vi "template_Job (JKI-SM).vi"() -> ()   [LabVIEW 2013]
doc: "Job template based on the popular JKI State Machine."
uses:
  <vilib>/LabVIEW Open Source Project/Cron Scheduler/Job/Job.lvclass
  <vilib>/LabVIEW Open Source Project/Cron Scheduler/Job/Job.lvclass/Job.ctl
  <vilib>/LabVIEW Open Source Project/Cron Scheduler/Job/Read Abort Notifier.vi
panel:
  out "Job out":refnum<class "Job.lvclass">
  out "error out":errorcluster
  in  "Job":refnum<class "Job.lvclass">
  out "stdout":string
  in  "stdin":string
  # "Macro: Initialize\nList the tasks to be execute for this job\n\nThere are two ways to terminate the job: \n1- Call the \"Macro: Exit\" state at the end of your task execution.\n2- Comment out the \"Macro: Exit\" state in \"Macro: Initialize\" case and monitor a Job completion condition instead. Use the \"Action: Check Job Complete\" state to instruct the job to terminate.\n\nAction: Read Standard Input\nUse this case to read the stdin terminal and initialize your job.\n\nAction: Write Standard Output\nMake sure to write your return value to the stdout terminal before exiting this VI."
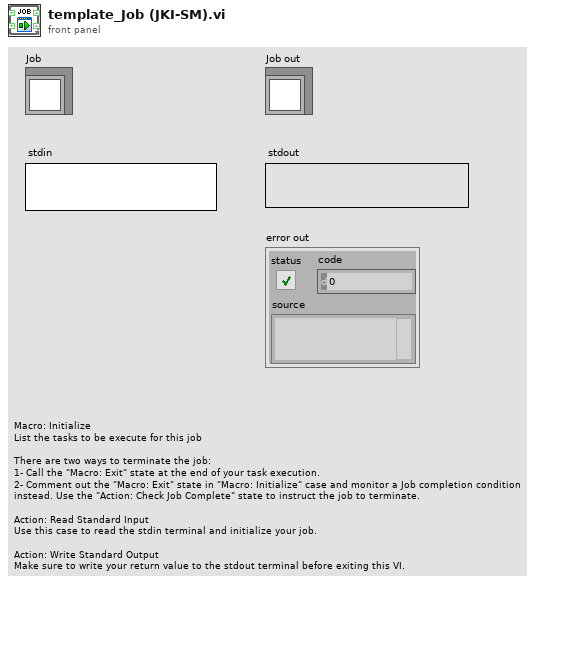
[diagram p1: front panel]
types:
  T1 = enum32{"Invalid", "Standard", "Closed", "Hidden", "Minimized", "Maximized"}
  T2 = enum32{"invalid app kind", "Development System", "Run Time System", "Student Edition", "Embedded LabVIEW", "Evaluation", "Custom"}
  T3 = cluster{"Core":cluster{"Current VI Reference":refnum<vi>, "Close Panel on Exit?":bool}, "Job":refnum<class "Job.lvclass">, "stdin":string, "stdout":string, "stderror":errorcluster, "start time":timestamp}
  T4 = cluster{"Current VI Reference":refnum<vi>, "Close Panel on Exit?":bool}
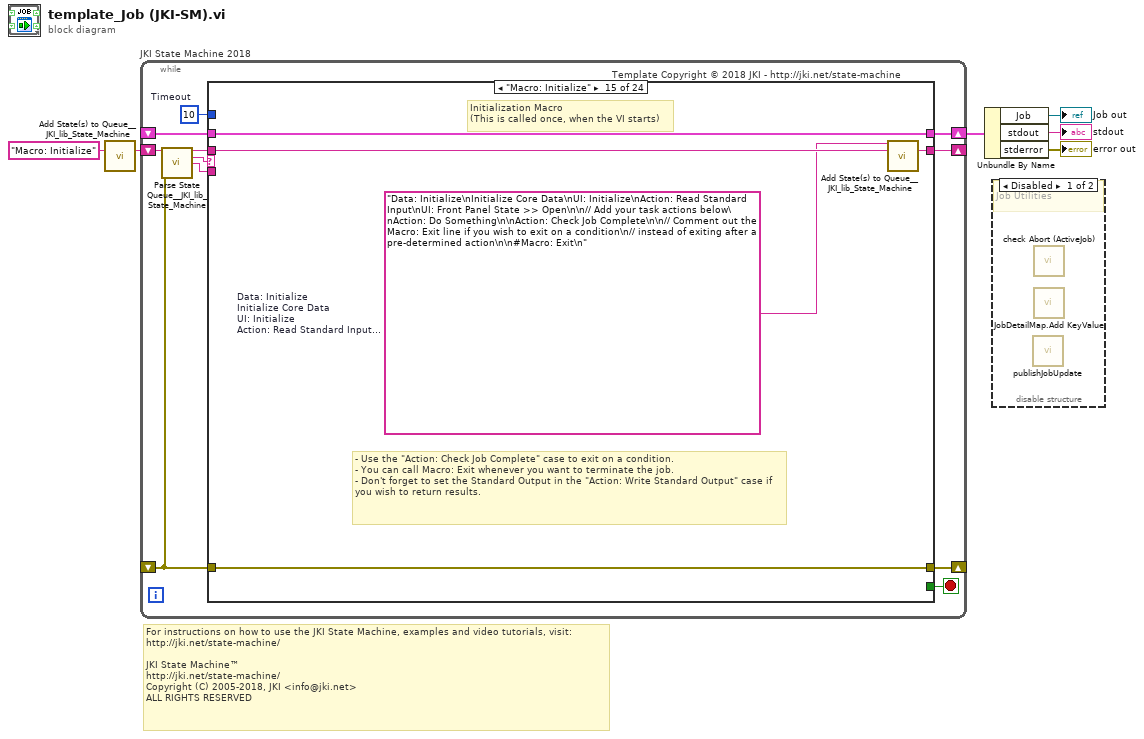
[diagram p0: block diagram]
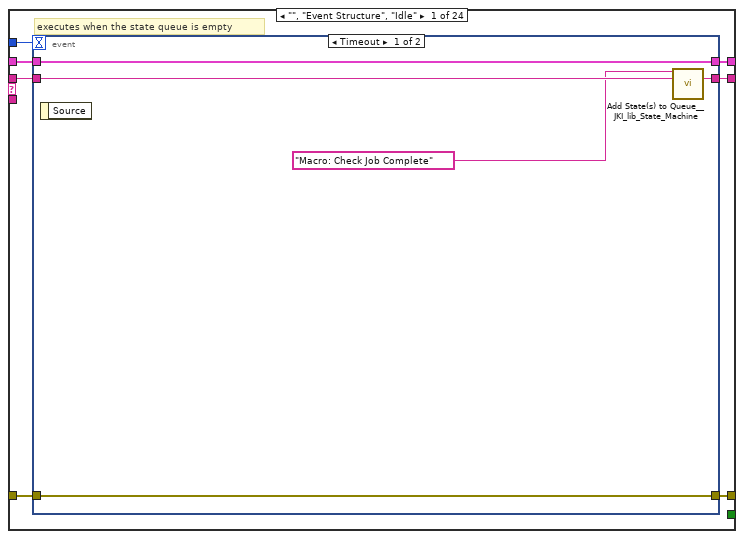
[diagram p3: hidden frame]
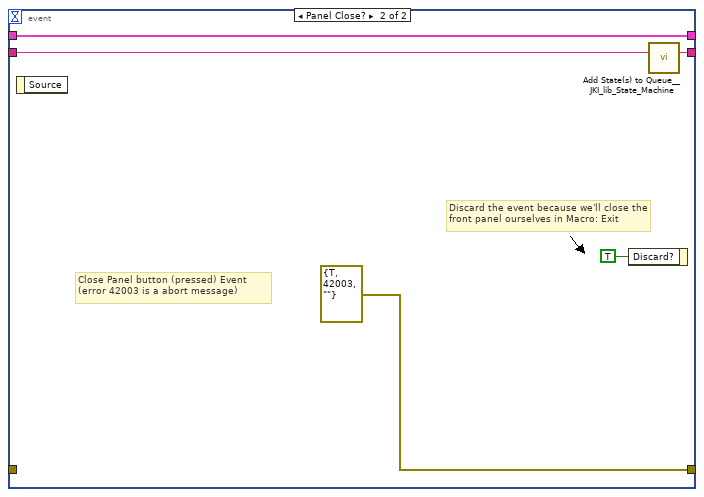
[diagram p4: hidden frame]
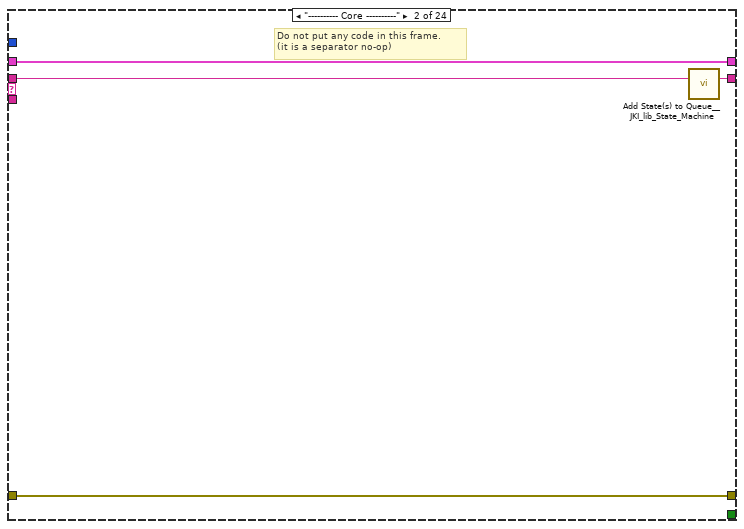
[diagram p5: hidden frame]
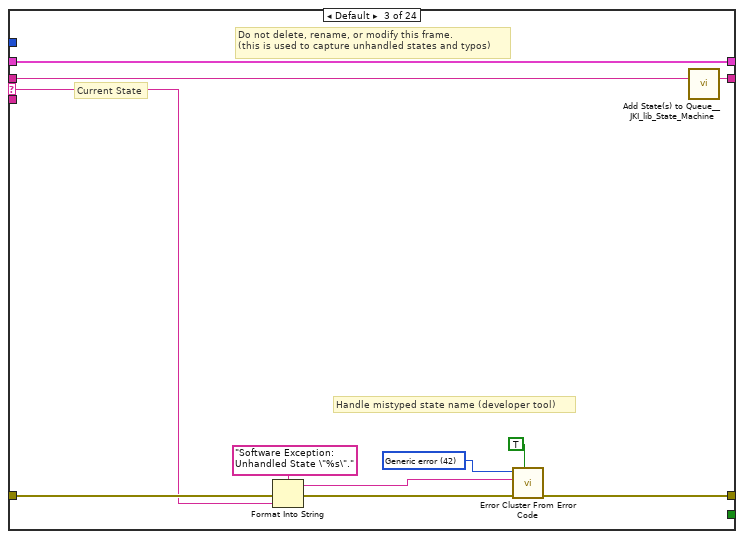
[diagram p6: hidden frame]
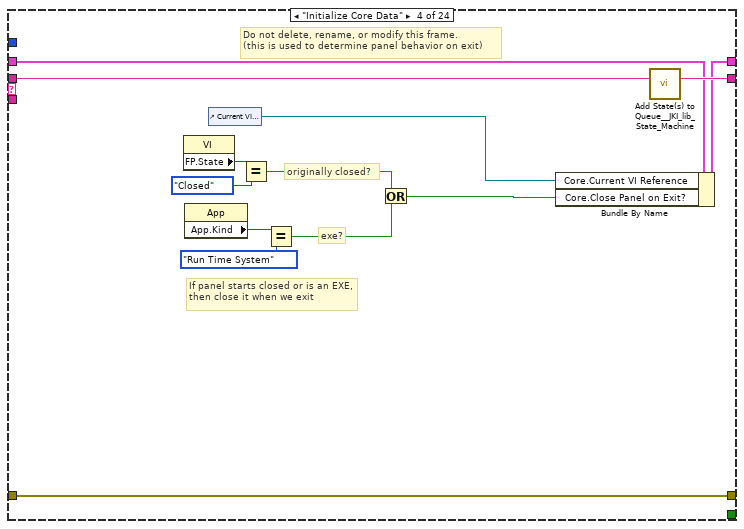
[diagram p7: hidden frame]
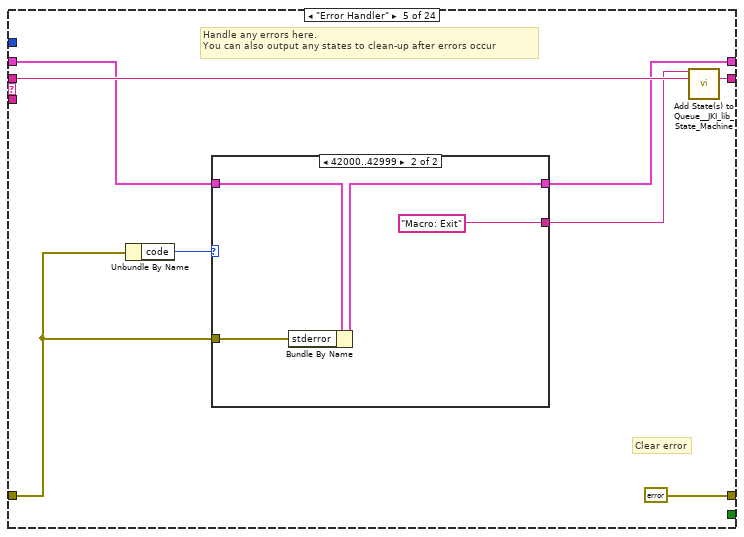
[diagram p8: hidden frame]
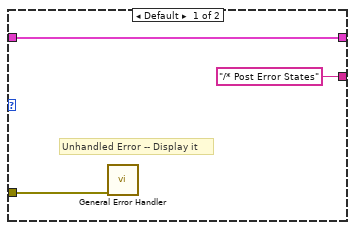
[diagram p9: hidden frame]
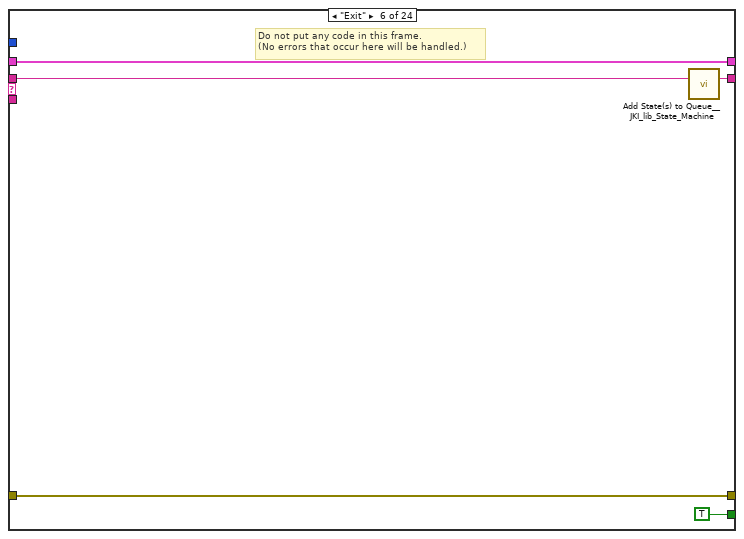
[diagram p10: hidden frame]
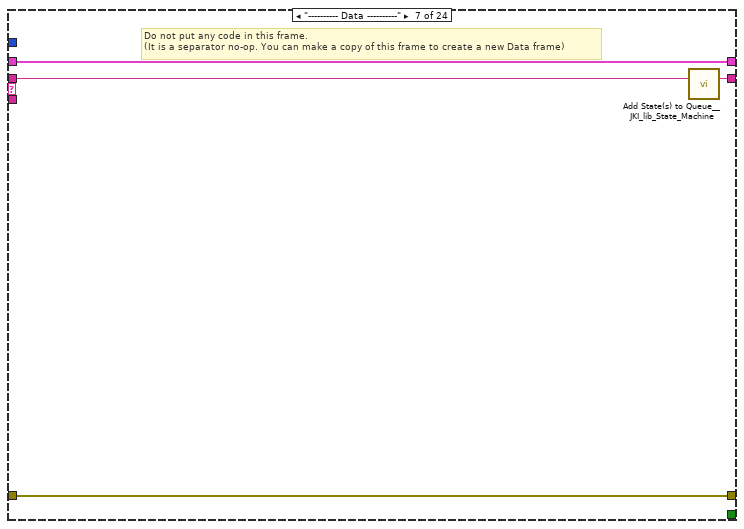
[diagram p11: hidden frame]
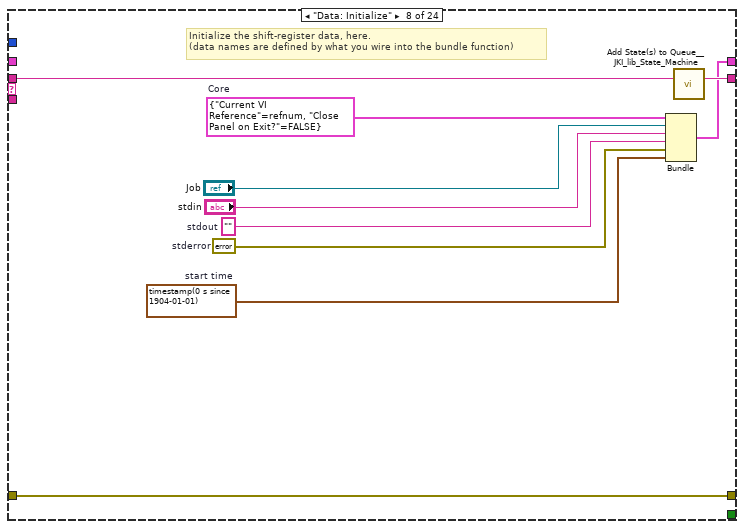
[diagram p12: hidden frame]
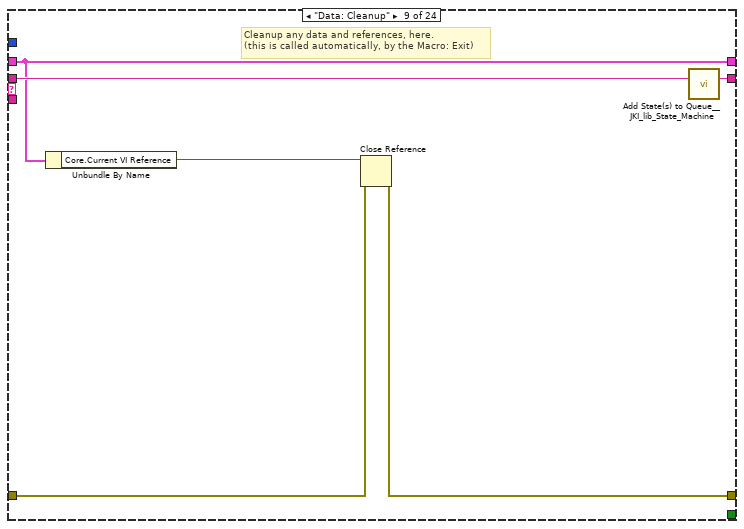
[diagram p13: hidden frame]
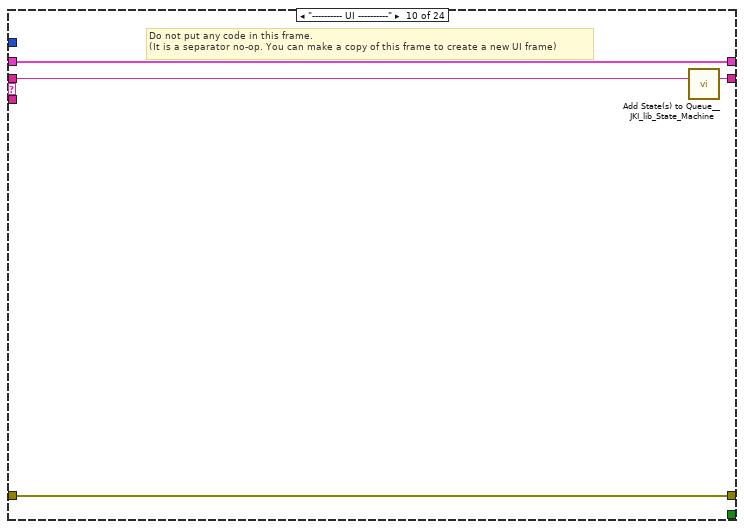
[diagram p14: hidden frame]
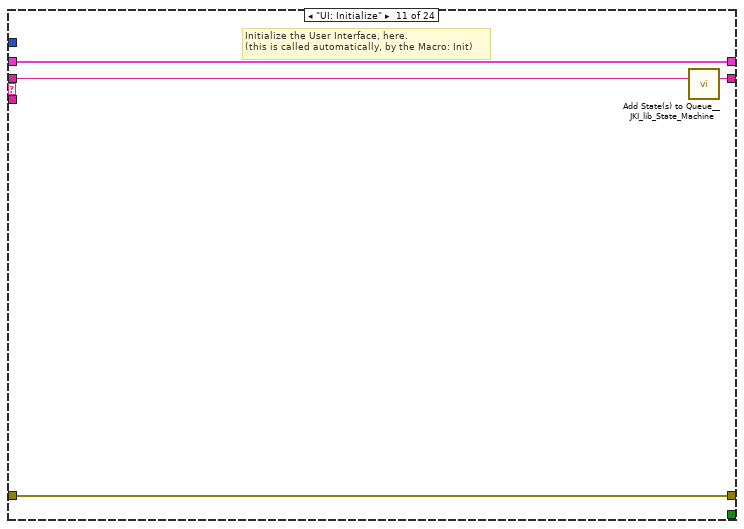
[diagram p15: hidden frame]
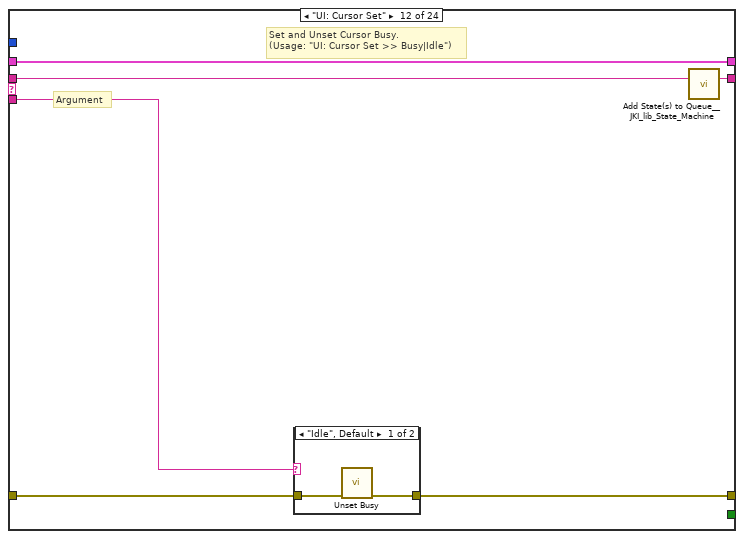
[diagram p16: hidden frame]
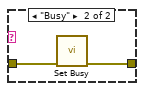
[diagram p17: hidden frame]
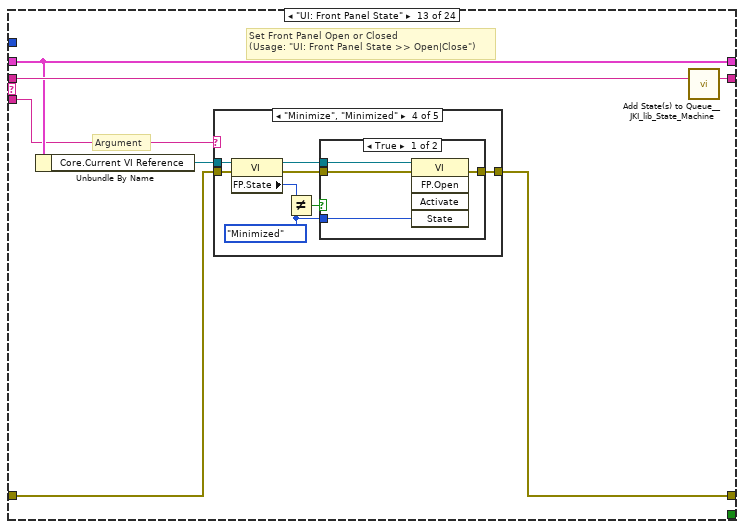
[diagram p18: hidden frame]
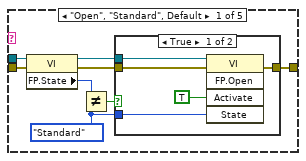
[diagram p19: hidden frame]
diagram:
  # "For instructions on how to use the JKI State Machine, examples and video tutorials, visit:\nhttp://jki.net/state-machine/\n\nJKI State Machine™\nhttp://jki.net/state-machine/\nCopyright (C) 2005-2018, JKI <info@jki.net>\nALL RIGHTS RESERVED"
  n1 = call <vilib>:"Add State(s) to Queue__JKI_lib_State_Machine.vi"("State(s) in (\"\")"="Macro: Initialize") -> ("States Out"=w6:string)  [unwired: 14 in]
  n2 = while "JKI State Machine 2018" {
    shift-right: [w10] -> w4
    shift-left: _ -> [w9]
    shift-right: [w13] -> _
    shift-left: _ -> [w7]
    shift-right: [w12] -> _
    shift-left: w6 -> [w14]
    stop <- w11 stop-if-true
    w8 = 10  # Timeout
    # "Template Copyright © 2018 JKI - http://jki.net/state-machine"
    n3 = call <vilib>:"Parse State Queue__JKI_lib_State_Machine.vi"("State Queue"=w14, "Error In (no error)"=w7) -> ("Remaining States"=w16:string, "Current State"=w17:string, "Arguments"=w15:string)  [unwired: 11 in]
    n4 = case shown="\"Macro: Initialize\"" w17 {
      selector: w17 -> [_ _ w39 _ _ _ _ _ _ _ _ _ _ _ _ _ _ _ w230 _ _ _ _ _]
      tunnel: w16 -> [w24 w38 w43 w62 w70 w82 w86 w96 w102 w106 w110 w116 w127 w196 w201 w206 w217 w223 w236 w251 w261 w271 w277 w288]
      tunnel: w15 -> [_ _ _ _ _ _ _ _ _ _ _ w111 w121 _ _ _ _ _ _ _ _ _ _ _]
      tunnel: w9 -> [w22 w35 w41 w55 w65 w80 w83 _ w97 w103 w108 w114 w123 w193 w198 w203 w214 w220 w234 w243 w259 w269 w273 w280]
      tunnel: [w21 w36 w45 w59 errorcluster {"status"=FALSE, "code"=0, "source"=""} ("error out") w79 w84 w93 w98 w104 w107 w112 w124 w194 w199 w204 w215 w221 w225 w249 w255 w263 w275 w286] -> w13
      tunnel: w7 -> [w20 w36 w44 w59 w66 w79 w84 w93 w99 w104 w107 w113 w125 w194 w199 w204 w215 w221 w231 w249 w252 w264 w275 w286]
      tunnel: [w23 w37 w42 w61 w69 w81 w85 w95 w101 w105 w109 w115 w126 w195 w200 w205 w216 w222 w235 w250 w260 w270 w276 w287] -> w12
      tunnel: [_ _ _ _ _ TRUE _ _ _ _ _ _ _ _ _ _ _ _ _ _ _ _ _ _] -> w11
      tunnel: [w19 w35 w41 w60 w64 w80 w83 w94 w97 w103 w108 w114 w123 w193 w198 w203 w214 w219 w233 w248 w258 w268 w272 w285] -> w10
      tunnel: w8 -> [w18 _ _ _ _ _ _ _ _ _ _ _ _ _ _ _ _ _ _ _ _ _ _ _]
      frame "", "Event Structure", "Idle" {
        # "executes when the state queue is empty"
        n5 = event shown="[0] Timeout" {
          selector: _ -> [_ _]
          dyn-events: _ -> [_ _]
          timeout: w18 -> [_ _]
          tunnel: w24 -> [w29 w34]
          tunnel: [w28 w33] -> w23
          tunnel: w22 -> [w26 w32]
          tunnel: [w27 errorcluster {"status"=TRUE, "code"=42003, "source"=""} ("error constant")] -> w21
          tunnel: w20 -> [w27 _]
          tunnel: [w26 w32] -> w19
          event Timeout {
            n6 = event-data() -> ()  [unwired: 1 in, 1 out]
            n7 = call <vilib>:"Add State(s) to Queue__JKI_lib_State_Machine.vi"("State(s) in Front (\"\")"="Macro: Check Job Complete", "State(s) in (\"\")"=w29) -> ("States Out"=w28:string)  [unwired: 13 in]
          }
          event Panel Close? {
            # "Discard the event because we'll close the front panel ourselves in Macro: Exit"
            # "Close Panel button (pressed) Event\n(error 42003 is a abort message)"
            n8 = event-data() -> ()  [unwired: 1 in, 1 out]
            n9 = event-data("Discard?"=TRUE) -> ()  [unwired: 1 in, 1 out]
            n10 = call <vilib>:"Add State(s) to Queue__JKI_lib_State_Machine.vi"("State(s) in (\"\")"=w34) -> ("States Out"=w33:string)  [unwired: 14 in]
          }
        }
      }
      frame "---------- Core ----------" {
        # "Do not put any code in this frame.\n(it is a separator no-op)"
        n11 = call <vilib>:"Add State(s) to Queue__JKI_lib_State_Machine.vi"("State(s) in (\"\")"=w38) -> ("States Out"=w37:string)  [unwired: 14 in]
      }
      frame Default {
        w48 = 42 items=["No error", "Argument error", "Memory is full", "Out of zone", "End of file", "File already open", "Generic file I/O error", "File not found", "File permission error", "Disk is full", "Duplicate path", "Too many files open", "System feature not enabled", "Resource file not found", "Cannot add resource", "Resource not found", "Image not found", "Image memory error", "Pen does not exist", "Config type invalid", "Config token not found", "Config parse error", "Config memory error", "Bad external code format", "Bad external code offset", "External code not present", "Null window", "Destroy window error", "Null menu", "Print aborted", "Bad print record", "Print driver error", "Windows error during printing", "Memory error during printing", "Print dialog error", "Generic print error", "Invalid device refnum", "Device not found", "Device parameter error", "Device unit error", "Cannot open device", "Device call aborted", "Generic error", "Cancelled by user", "Object ID too low", "Object ID too high", "Object not in heap", "Unknown heap", "Unknown object (invalid DefProc)", "Unknown object (DefProc not in table)", "Message out of range", "Invalid (null) method", "Unknown message", "Manager call not supported", "Bad address", "Network operation in progress", "Network operation timed out", "Connection is busy", "Network attribute not supported", "Network error", "Address in use", "System out of memory", "Connection aborted", "Connection refused", "Not connected", "Already connected", "Connection closed", "Initialization error (interapplication manager)", "Bad occurrence", "Wait on unbound occurrence handler", "Occurrence queue overflow", "Datalog type conflict", "Unused", "Unrecognized type (interapplication manager)", "Memory corrupt", "Failed to make temporary DLL", "Old CIN version", "Drag socket not found", "Failed to load drop-object", "Failed to register OLE object", "Failed to release OLE object", "Format specifier type mismatch", "Unknown format specifier", "Too few format specifiers", "Too many format specifiers", "Scan failed", "Newer CIN version", "Error converting to variant", "Runtime menu error", "Password tampered", "Variant attribute not found", "Incompatible variant data type", "Event data is not available", "Event Store is not present", "Occurrence is not found", "Event Queue is not created", "Event info is not available", "Refnum passed is NULL", "Error retrieving Class GUID", "Error retrieving CoClass GUID", "Error retrieving TypeLib GUID.", "Bad built application magic bytes.", "Specific driver is different from the specific driver associated with the Logical Name.", "There is no session opened to the class driver.", "Max Error", "MAX - Error with config objects", "MAX - Error loading configuration", "MAX - Group not supported"]
        # "Current State"
        # "Do not delete, rename, or modify this frame.\n(this is used to capture unhandled states and typos)"
        # "Handle mistyped state name (developer tool)"
        n12 = Format Into String(format string="Software Exception: Unhandled State \"%s\"." ("message"), error in=w44, w39) -> (resulting string=w47:string, error out=w46:errorcluster)  [unwired: 1 in]
        n13 = call <vilib>:"Error Cluster From Error Code.vi"("show call chain? (False)"=TRUE, "error in (no error)"=w46, "error message (\"\")"=w47, "error code (0)"=w48) -> ("error out"=w45:errorcluster)  [unwired: 5 in]
        n14 = call <vilib>:"Add State(s) to Queue__JKI_lib_State_Machine.vi"("State(s) in (\"\")"=w43) -> ("States Out"=w42:string)  [unwired: 14 in]
      }
      frame "Initialize Core Data" {
        # "Do not delete, rename, or modify this frame.\n(this is used to determine panel behavior on exit)"
        # "originally closed?"
        # "exe?"
        # "If panel starts closed or is an EXE, then close it when we exit"
        n15 = property class="VI"() -> ("FP.State"=w52:T1)  [unwired: 2 in, 2 out]
        n16 = property class="App"() -> ("App.Kind"=w58:T2)  [unwired: 2 in, 2 out]
        n17 = control-ref of="Current VI Reference"() -> (w53:refnum<vi>)
        n18 = Equal?(x=w52, y=T1."Closed" ("Front Panel Window:State")) -> (x = y?=w50:bool)
        n19 = Equal?(x=w58, y=T2."Run Time System" ("Application:Kind")) -> (x = y?=w56:bool)
        n20 = Or(x=w50, y=w56) -> (x .or. y?=w54:bool)
        n21 = Bundle By Name(cluster=w55, "Core.Current VI Reference"=w53, "Core.Close Panel on Exit?"=w54) -> (w60:T3)
        n22 = call <vilib>:"Add State(s) to Queue__JKI_lib_State_Machine.vi"("State(s) in (\"\")"=w62) -> ("States Out"=w61:string)  [unwired: 14 in]
      }
      frame "Error Handler" {
        # "Handle any errors here.\nYou can also output any states to clean-up after errors occur"
        # "Clear error"
        n23 = Unbundle By Name(w66) -> ("code"=w67:i32)
        n24 = case shown="42000..42999" w67 {
          tunnel: w66 -> [w73 w76]
          tunnel: w65 -> [w72 w77]
          tunnel: [w72 w75] -> w64
          tunnel: ["/* Post Error States" "Macro: Exit"] -> w63
          frame Default {
            # "Unhandled Error -- Display it"
            n25 = call <vilib>:"General Error Handler.vi"("error in (no error)"=w73) -> ()  [unwired: 10 in, 5 out]
          }
          frame 42000..42999 {
            n26 = Bundle By Name(cluster=w77, "stderror"=w76) -> (w75:T3)
          }
        }
        n27 = call <vilib>:"Add State(s) to Queue__JKI_lib_State_Machine.vi"("State(s) in Front (\"\")"=w63, "State(s) in (\"\")"=w70) -> ("States Out"=w69:string)  [unwired: 13 in]
      }
      frame "Exit" {
        # "Do not put any code in this frame.\n(No errors that occur here will be handled.)"
        n28 = call <vilib>:"Add State(s) to Queue__JKI_lib_State_Machine.vi"("State(s) in (\"\")"=w82) -> ("States Out"=w81:string)  [unwired: 14 in]
      }
      frame "---------- Data ----------" {
        # "Do not put any code in this frame.\n(It is a separator no-op. You can make a copy of this frame to create a new Data frame)"
        n29 = call <vilib>:"Add State(s) to Queue__JKI_lib_State_Machine.vi"("State(s) in (\"\")"=w86) -> ("States Out"=w85:string)  [unwired: 14 in]
      }
      frame "Data: Initialize" {
        w87 = timestamp(0 s since 1904-01-01)  # start time
        w88 = errorcluster {"status"=FALSE, "code"=0, "source"=""}  # stderror
        w89 = ""  # stdout
        w92 = T4 {"Current VI Reference"=refnum, "Close Panel on Exit?"=FALSE}  # Core
        # "Initialize the shift-register data, here.\n(data names are defined by what you wire into the bundle function)"
        n30 = Bundle("Core"=w92, "Job"="Job", "stdin"="stdin", "stdout"=w89, "stderror"=w88, "start time"=w87) -> (w94:T3)  [unwired: 1 in]
        n31 = call <vilib>:"Add State(s) to Queue__JKI_lib_State_Machine.vi"("State(s) in (\"\")"=w96) -> ("States Out"=w95:string)  [unwired: 14 in]
      }
      frame "Data: Cleanup" {
        # "Cleanup any data and references, here.\n(this is called automatically, by the Macro: Exit)"
        n32 = Unbundle By Name(w97) -> ("Core.Current VI Reference"=w100:refnum<vi>)
        n33 = Close Reference(reference=w100, error in (no error)=w99) -> (error out=w98:errorcluster)
        n34 = call <vilib>:"Add State(s) to Queue__JKI_lib_State_Machine.vi"("State(s) in (\"\")"=w102) -> ("States Out"=w101:string)  [unwired: 14 in]
      }
      frame "---------- UI ----------" {
        # "Do not put any code in this frame.\n(It is a separator no-op. You can make a copy of this frame to create a new UI frame)"
        n35 = call <vilib>:"Add State(s) to Queue__JKI_lib_State_Machine.vi"("State(s) in (\"\")"=w106) -> ("States Out"=w105:string)  [unwired: 14 in]
      }
      frame "UI: Initialize" {
        # "Initialize the User Interface, here.\n(this is called automatically, by the Macro: Init)"
        n36 = call <vilib>:"Add State(s) to Queue__JKI_lib_State_Machine.vi"("State(s) in (\"\")"=w110) -> ("States Out"=w109:string)  [unwired: 14 in]
      }
      frame "UI: Cursor Set" {
        # "Argument"
        # "Set and Unset Cursor Busy.\n(Usage: \"UI: Cursor Set >> Busy|Idle\")"
        n37 = case shown="\"Idle\", Default" w111 {
          tunnel: w113 -> [w118 w120]
          tunnel: [w117 w119] -> w112
          frame "Idle", Default {
            n38 = call <vilib>:"Unset Busy.vi"("error in (no error)"=w118) -> ("error out"=w117:errorcluster)  [unwired: 10 in]
          }
          frame "Busy" {
            n39 = call <vilib>:"Set Busy.vi"("error in (no error)"=w120) -> ("error out"=w119:errorcluster)  [unwired: 9 in, 1 out]
          }
        }
        n40 = call <vilib>:"Add State(s) to Queue__JKI_lib_State_Machine.vi"("State(s) in (\"\")"=w116) -> ("States Out"=w115:string)  [unwired: 14 in]
      }
      frame "UI: Front Panel State" {
        # "Argument"
        # "Set Front Panel Open or Closed\n(Usage: \"UI: Front Panel State >> Open|Close\")"
        n41 = Unbundle By Name(w123) -> ("Core.Current VI Reference"=w122:refnum<vi>)
        n42 = case shown="\"Minimize\", \"Minimized\"" w121 {
          tunnel: w125 -> [w133 w148 w159 w172 w185]
          tunnel: [w135 w149 w161 w174 w187] -> w124
          tunnel: w122 -> [w134 w146 w160 w173 w186]
          frame "Open", "Standard", Default {
            w128 = T1."Standard" ("State")
            n43 = property class="VI"(reference=w134, error in=w133) -> (reference out=w131:refnum<vi>, error out=w132:errorcluster, "FP.State"=w130:T1)
            n44 = Not Equal?(x=w130, y=w128) -> (x != y?=w129:bool)
            n45 = case shown="True" w129 {
              tunnel: [w139 w141] -> w135
              tunnel: w132 -> [w138 w141]
              tunnel: w131 -> [w137 _]
              tunnel: w128 -> [w136 _]
              frame True {
                n46 = invoke class="VI" method="FP.Open"(reference=w137, error in=w138, "Activate"=TRUE, "State"=w136) -> (error out=w139:errorcluster)  [unwired: 1 in, 4 out]
              }
              frame False {
              }
            }
          }
          frame "Close", "Closed" {
            n47 = property class="VI"(reference=w146, error in=w148) -> (reference out=w145:refnum<vi>, error out=w147:errorcluster, "FP.State"=w143:T1)
            n48 = Not Equal?(x=w143, y=T1."Closed" ("Front Panel Window:State")) -> (x != y?=w142:bool)
            n49 = case shown="True" w142 {
              tunnel: [w150 w153] -> w149
              tunnel: w147 -> [w150 w152]
              tunnel: w145 -> [_ w151]
              frame False {
              }
              frame True {
                n50 = invoke class="VI" method="FP.Close"(reference=w151, error in=w152) -> (error out=w153:errorcluster)  [unwired: 1 in, 2 out]
              }
            }
          }
          frame "Hidden", "Hide" {
            w154 = T1."Hidden" ("State")
            n51 = property class="VI"(reference=w160, error in=w159) -> (reference out=w157:refnum<vi>, error out=w158:errorcluster, "FP.State"=w156:T1)
            n52 = Not Equal?(x=w156, y=w154) -> (x != y?=w155:bool)
            n53 = case shown="True" w155 {
              tunnel: [w165 w166] -> w161
              tunnel: w158 -> [w164 w166]
              tunnel: w157 -> [w163 _]
              tunnel: w154 -> [w162 _]
              frame True {
                n54 = invoke class="VI" method="FP.Open"(reference=w163, error in=w164, "State"=w162) -> (error out=w165:errorcluster)  [unwired: 2 in, 4 out]
              }
              frame False {
              }
            }
          }
          frame "Minimize", "Minimized" {
            w167 = T1."Minimized" ("State")
            n55 = property class="VI"(reference=w173, error in=w172) -> (reference out=w170:refnum<vi>, error out=w171:errorcluster, "FP.State"=w169:T1)
            n56 = Not Equal?(x=w169, y=w167) -> (x != y?=w168:bool)
            n57 = case shown="True" w168 {
              tunnel: [w178 w179] -> w174
              tunnel: w171 -> [w177 w179]
              tunnel: w170 -> [w176 _]
              tunnel: w167 -> [w175 _]
              frame True {
                n58 = invoke class="VI" method="FP.Open"(reference=w176, error in=w177, "State"=w175) -> (error out=w178:errorcluster)  [unwired: 2 in, 4 out]
              }
              frame False {
              }
            }
          }
          frame "Maximize", "Maximized" {
            w180 = T1."Maximized" ("State")
            n59 = property class="VI"(reference=w186, error in=w185) -> (reference out=w183:refnum<vi>, error out=w184:errorcluster, "FP.State"=w182:T1)
            n60 = Not Equal?(x=w182, y=w180) -> (x != y?=w181:bool)
            n61 = case shown="True" w181 {
              tunnel: [w191 w192] -> w187
              tunnel: w184 -> [w190 w192]
              tunnel: w183 -> [w189 _]
              tunnel: w180 -> [w188 _]
              frame True {
                n62 = invoke class="VI" method="FP.Open"(reference=w189, error in=w190, "State"=w188) -> (error out=w191:errorcluster)  [unwired: 2 in, 4 out]
              }
              frame False {
              }
            }
          }
        }
        n63 = call <vilib>:"Add State(s) to Queue__JKI_lib_State_Machine.vi"("State(s) in (\"\")"=w127) -> ("States Out"=w126:string)  [unwired: 14 in]
      }
      frame "---------- Macro ----------" {
        # "Do not put any code in this frame.\n(It is a separator no-op. You can make a copy of this frame to create a new Macro frame)"
        n64 = call <vilib>:"Add State(s) to Queue__JKI_lib_State_Machine.vi"("State(s) in (\"\")"=w196) -> ("States Out"=w195:string)  [unwired: 14 in]
      }
      frame "Macro: Initialize" {
        w197 = "Data: Initialize\nInitialize Core Data\nUI: Initialize\nAction: Read Standard Input\nUI: Front Panel State >> Open\n\n// Add your task actions below\nAction: Do Something\n\nAction: Check Job Complete\n\n// Comment out the Macro: Exit line if you wish to exit on a condition\n// instead of exiting after a pre-determined action\n\n#Macro: Exit\n"  # Data: Initialize Initialize Core Data UI: Initialize Action: Read Standard Input UI: Front Panel State >> Open  // Add your task actions below Action: Do Something  Action: Check Job Complete  // Comment out the Macro: Exit line if you wish to exit on a condition // instead of exiting after a pre-determined action  #Macro: Exit
        # "- Use the \"Action: Check Job Complete\" case to exit on a condition.\n- You can call Macro: Exit whenever you want to terminate the job.\n- Don't forget to set the Standard Output in the \"Action: Write Standard Output\" case if you wish to return results."
        # "Initialization Macro\n(This is called once, when the VI starts)"
        n65 = call <vilib>:"Add State(s) to Queue__JKI_lib_State_Machine.vi"("State(s) in Front (\"\")"=w197, "State(s) in (\"\")"=w201) -> ("States Out"=w200:string)  [unwired: 13 in]
      }
      frame "Macro: Check Job Complete" {
        # "Job Monitoring Macro\n(This is called regularly when the UI is idle)"
        n66 = call <vilib>:"Add State(s) to Queue__JKI_lib_State_Machine.vi"("State(s) in Front (\"\")"="Action: Check Job Complete\nAction: Check Abort", "State(s) in (\"\")"=w206) -> ("States Out"=w205:string)  [unwired: 13 in]
      }
      frame "Macro: Exit" {
        # "Exit Macro\n(This is called once, when the VI exits)"
        n67 = Unbundle By Name(w214) -> ("Core.Close Panel on Exit?"=w213:bool)
        n68 = Select(t="UI: Front Panel State >> Close", s=w213, f="") -> (s? t:f=w210:string)
        n69 = call <vilib>:"Add State(s) to Queue__JKI_lib_State_Machine.vi"("State(s) in Front (\"\")"="Action: Write Standard Output", "State(s) in (\"\")"=w210, "State(s) at Back (\"\")"="Data: Cleanup\nExit") -> ("States Out"=w208:string)  [unwired: 12 in]
        n70 = call <vilib>:"Add State(s) to Queue__JKI_lib_State_Machine.vi"("State(s) in Front (\"\")"=w208, "State(s) in (\"\")"=w217) -> ("States Out"=w216:string)  [unwired: 13 in]
      }
      frame "---------- Action ----------" {
        # "Action Separator\n(You can make a copy of, or modify, this frame)"
        n71 = Unbundle By Name(w220) -> ("Job"=w218:refnum<class "Job.lvclass">)  [unwired: 1 out]
        n72 = Bundle By Name(cluster=w220, "Job"=w218) -> (w219:T3)
        n73 = call <vilib>:"Add State(s) to Queue__JKI_lib_State_Machine.vi"("State(s) in (\"\")"=w223) -> ("States Out"=w222:string)  [unwired: 14 in]
      }
      frame "Action: Do Something" {
        # "Update Status"
        # "Add custom data\nto the job report"
        n74 = Unbundle By Name(w234) -> ("Job"=w232:refnum<class "Job.lvclass">)  [unwired: 1 out]
        n75 = stacked-sequence {
          tunnel: [w237] -> w229
          frame #0 {
            # "Perform an action"
            n76 = Random Number (0-1)() -> (number: 0 to 1=w237:dbl)
          }
        }
        n77 = call <vilib>:"JobDetailMap.Add KeyValue.vi"("error in (no error)"=w231, "Value"=w229, "Key"=w230, "Job in"=w232) -> ("error out"=w226:errorcluster, "Job out"=w228:refnum<class "Job.lvclass">)  [unwired: 6 in]
        n78 = call <vilib>:"publishJobUpdate.vi"("error in (no error)"=w226, "Status Message"="Status Update Message", "Job in"=w228) -> ("error out"=w225:errorcluster, "Job out"=w227:refnum<class "Job.lvclass">)  [unwired: 7 in]
        n79 = Bundle By Name(cluster=w234, "Job"=w227) -> (w233:T3)
        n80 = call <vilib>:"Add State(s) to Queue__JKI_lib_State_Machine.vi"("State(s) in (\"\")"=w236) -> ("States Out"=w235:string)  [unwired: 14 in]
      }
      frame "Action: Check Job Complete" {
        # "Terminates after a delay (demo).\nReplace with your own condition."
        n81 = Unbundle By Name(w243) -> ("Job"=w247:refnum<class "Job.lvclass">)
        n82 = Unbundle By Name(w243) -> ("start time"=w241:timestamp)
        n83 = Get Date/Time In Seconds() -> (seconds since 1Jan1904=w242:timestamp)
        n84 = Subtract(x=w242, y=w241) -> (x-y=w240:dbl)
        n85 = Bundle By Name(cluster=w243, "Job"=w247) -> (w248:T3)
        n86 = Greater Or Equal?(x=w240, y=3.0) -> (x >= y?=w238:bool)
        n87 = Select(t="Macro: Exit", s=w238, f="") -> (s? t:f=w244:string)
        n88 = call <vilib>:"Add State(s) to Queue__JKI_lib_State_Machine.vi"("State(s) in Front (\"\")"=w244, "State(s) in (\"\")"=w251) -> ("States Out"=w250:string)  [unwired: 13 in]
      }
      frame "Action: Check Abort" {
        n89 = Unbundle By Name(w259) -> ("Job"=w254:refnum<class "Job.lvclass">)  [unwired: 1 out]
        n90 = call <vilib>:"check Abort (ActiveJob).vi"("error in (no error)"=w252, "Job in"=w254) -> ("error out"=w256:errorcluster, "Abort"=w257:bool, "Job out"=w253:refnum<class "Job.lvclass">)  [unwired: 6 in, 1 out]
        n91 = Bundle By Name(cluster=w256, "status"=w257) -> (w255:errorcluster)
        n92 = Bundle By Name(cluster=w259, "Job"=w253) -> (w258:T3)
        n93 = call <vilib>:"Add State(s) to Queue__JKI_lib_State_Machine.vi"("State(s) in (\"\")"=w261) -> ("States Out"=w260:string)  [unwired: 14 in]
      }
      frame "Action: Update Map Data" {
        # "Use this pattern to add\nkey value pair data to the\nJob's map. This data is going\nto be available by the scheduler\nupon completion of the job."
        n94 = Unbundle By Name(w269) -> ("Job"=w267:refnum<class "Job.lvclass">)  [unwired: 1 out]
        n95 = Random Number (0-1)() -> (number: 0 to 1=w262:dbl)
        n96 = call <vilib>:"JobDetailMap.Add KeyValue.vi"("error in (no error)"=w264, "Value"=w262, "Key"="Value", "Job in"=w267) -> ("error out"=w263:errorcluster, "Job out"=w266:refnum<class "Job.lvclass">)  [unwired: 6 in]
        n97 = Bundle By Name(cluster=w269, "Job"=w266) -> (w268:T3)
        n98 = call <vilib>:"Add State(s) to Queue__JKI_lib_State_Machine.vi"("State(s) in (\"\")"=w271) -> ("States Out"=w270:string)  [unwired: 14 in]
      }
      frame "Action: Read Standard Input" {
        n99 = Unbundle By Name(w273) -> ()  [unwired: 2 out]
        n100 = Get Date/Time In Seconds() -> (seconds since 1Jan1904=w274:timestamp)
        n101 = Bundle By Name(cluster=w273, "start time"=w274) -> (w272:T3)
        n102 = call <vilib>:"Add State(s) to Queue__JKI_lib_State_Machine.vi"("State(s) in (\"\")"=w277) -> ("States Out"=w276:string)  [unwired: 14 in]
      }
      frame "Action: Write Standard Output" {
        n103 = Unbundle By Name(w280) -> ("stderror"=w282:errorcluster)
        n104 = Unbundle By Name(w280) -> ("Job"=w279:refnum<class "Job.lvclass">)
        n105 = Unbundle By Name(w282) -> ("code"=w281:i32)
        n106 = call <vilib>:"Explain exception code.vi"("exception"=w281, "Job type"=w279) -> ("exception message"=w278:string)  [unwired: 7 in, 2 out]
        n107 = Select(t=w278, s=w282, f="OK") -> (s? t:f=w283:string)
        n108 = Bundle By Name(cluster=w280, "stdout"=w283) -> (w285:T3)
        n109 = call <vilib>:"Add State(s) to Queue__JKI_lib_State_Machine.vi"("State(s) in (\"\")"=w288) -> ("States Out"=w287:string)  [unwired: 14 in]
      }
    }
  }
  n110 = Unbundle By Name(w4) -> ("Job"=→"Job out":refnum<class "Job.lvclass">, "stdout"=→"stdout":string, "stderror"=→"error out":errorcluster)
  n111 = disable-structure shown="Disabled" {
    frame Disabled {
      # "Job Utilities"
      n112 = call <vilib>:"publishJobUpdate.vi"() -> ()  [unwired: 10 in, 2 out]
      n113 = call <vilib>:"check Abort (ActiveJob).vi"() -> ()  [unwired: 8 in, 4 out]
      n114 = call <vilib>:"JobDetailMap.Add KeyValue.vi"() -> ()  [unwired: 10 in, 2 out]
    }
    frame Enabled {
    }
  }
